vi "Online_target_rebooter.vi"   [LabVIEW 2021]
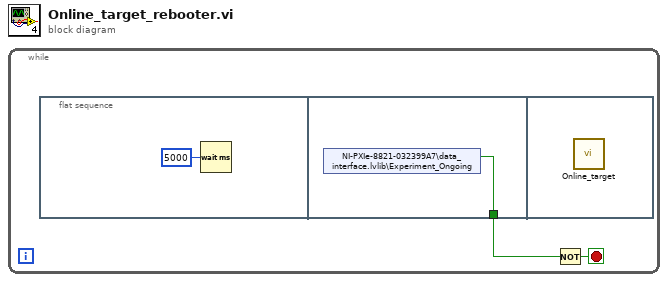
[diagram p0: block diagram]
diagram:
  n1 = while {
    stop <- w1 stop-if-true
    n2 = flat-sequence {
      tunnel: [w4] -> w2
      frame #0 {
        n3 = Wait (ms)(milliseconds to wait=u32 5000) -> ()  [unwired: 1 out]
      }
      frame #1 {
        n4 = shared-variable "NI-PXIe-8821-032399A7\\data_interface.lvlib\\Experiment_Ongoing"() -> (w4:bool)  [unwired: 1 in, 1 out]
      }
      frame #2 {
        n5 = call "Online_target.vi"() -> ()  [unwired: 12 in]
      }
    }
    n6 = Not(x=w2) -> (.not. x?=w1:bool)
  }
